vi "Get XCPCCP Master DB.vi"(8 "error in (no error)":errorcluster, 11 "Custom Device Node in":refnum<k24>) -> (0 "error out":errorcluster, 1 "file or folder exists?":bool, 2 "DB Path":path, 3 "Custom Device Node out":refnum<k24>)   [LabVIEW 2011]
uses:
  NationalInstruments.VeriStand.SystemStorage
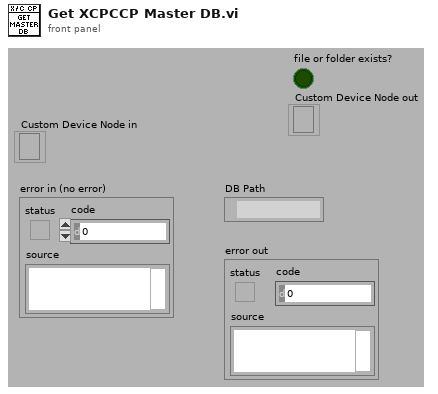
[diagram p1: front panel]
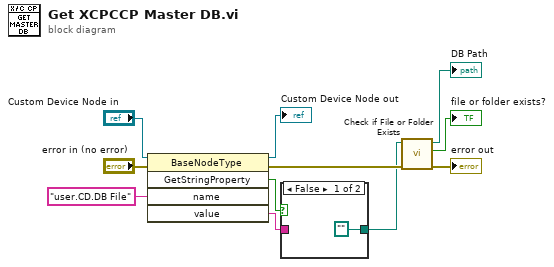
[diagram p0: block diagram]
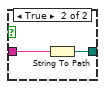
[diagram p2: hidden frame]
diagram:
  n1 = invoke class="BaseNodeType" method="GetStringProperty"(reference="Custom Device Node in", error in="error in (no error)", "name"="user.CD.DB File") -> (reference out=→"Custom Device Node out":refnum<k24>, error out=w5:errorcluster, "GetStringProperty"=w3:bool, "value"=w2:string)  [unwired: 2 in, 1 out]
  n2 = case shown="False" w3 {
    tunnel: w2 -> [_ w14]
    tunnel: [path "" w13] -> w1
    frame False {
    }
    frame True {
      n3 = String To Path(string=w14) -> (path=w13:path)
    }
  }
  n4 = call <vilib>:"Check if File or Folder Exists.vi"("error in (no error)"=w5, "path"=w1) -> ("error out"=→"error out":errorcluster, "file or folder exists?"=→"file or folder exists?":bool, "dup path"=→"DB Path":path)  [unwired: 7 in]
